vi "Read Tag Index.vi"(8 "error in (no error)":errorcluster, 11 "bt_Blackboard_Leaf Type in":refnum<class "bt_Blackboard_Leaf Type.lvclass">) -> (0 "error out":errorcluster, 2 "Tag Index":i32, 3 "bt_Blackboard_Leaf Type out":refnum<class "bt_Blackboard_Leaf Type.lvclass">)   [LabVIEW 2021, in "BT.lvlib" / "bt_Blackboard_Leaf Type.lvclass"]
uses:
  bt_Blackboard_Leaf Type.lvclass
  bt_Blackboard_Leaf Type.lvclass/bt_Blackboard_Leaf Type.ctl
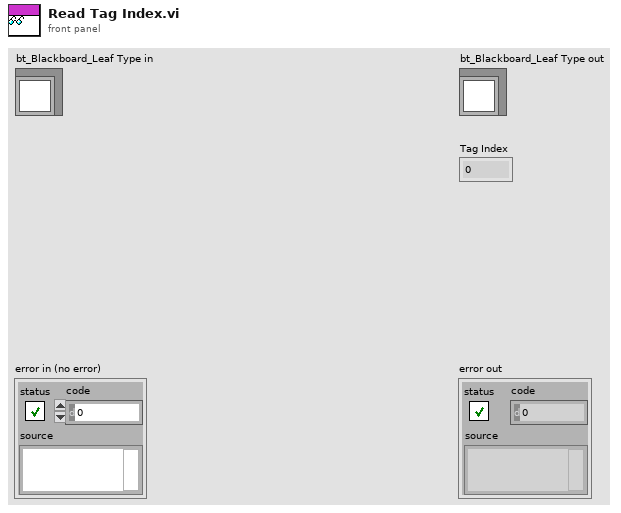
[diagram p1: front panel]
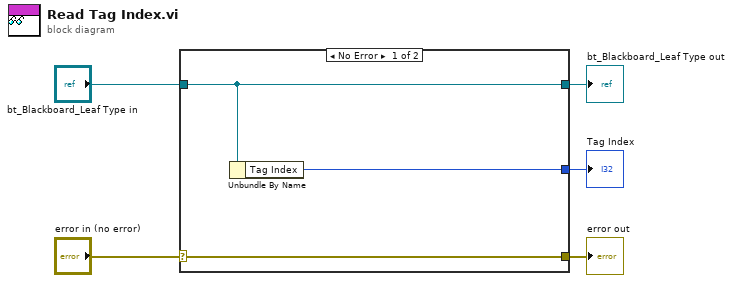
[diagram p0: block diagram]
diagram:
  n1 = case shown="No Error" "error in (no error)" {
    selector: "error in (no error)" -> [w8 w9]
    tunnel: [w8 w9] -> w4
    tunnel: [w7 w10] -> w2
    tunnel: "bt_Blackboard_Leaf Type in" -> [w7 w10]
    tunnel: [w6 _] -> w1
    frame No Error {
      n2 = Unbundle By Name(w7) -> ("Tag Index"=w6:i32)
    }
    frame Error {
    }
  }
  "error out" <- w4
  "bt_Blackboard_Leaf Type out" <- w2
  "Tag Index" <- w1
